vi "CreateSocketListener.vi"(0 "Universal Robot.lvclass in":refnum<class "Universal Robot.lvclass">, 5 "error in (no error)":errorcluster) -> (14 "Universal Robot.lvclass out":refnum<class "Universal Robot.lvclass">, 19 "error out":errorcluster)   [LabVIEW 2019, in "Universal Robot.lvclass"]
uses:
  Universal Robot.lvclass
  Universal Robot.lvclass/Universal Robot.ctl
  Client Interfaces/Socket Communication/Socket Communication.lvclass
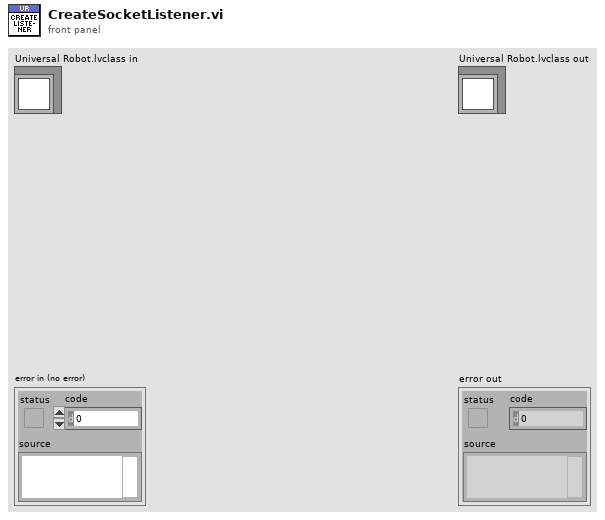
[diagram p1: front panel]
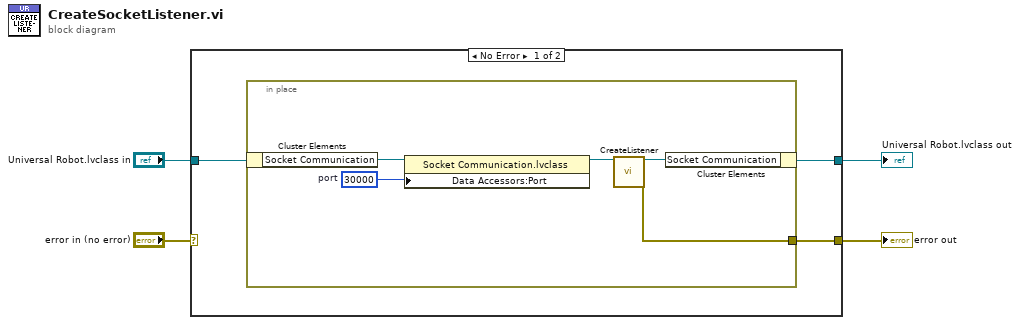
[diagram p0: block diagram]
diagram:
  n1 = case shown="No Error" "error in (no error)" {
    selector: "error in (no error)" -> [_ w14]
    tunnel: [w5 w14] -> w3
    tunnel: "Universal Robot.lvclass in" -> [w7 w13]
    tunnel: [w6 w13] -> w1
    frame No Error {
      n2 = in-place {
        in-place-border: [w9] -> w5
        w8 = u16 30000  # port
        n3 = in-place-cluster #1(w7) -> ("Socket Communication"=w12:refnum<class "Socket Communication.lvclass">)
        n4 = property class="Socket Communication.lvclass"(reference=w12, "Data Accessors:Port"=w8) -> (reference out=w11:refnum<class "Socket Communication.lvclass">)  [unwired: 1 in, 1 out]
        n5 = call "CreateListener.vi"("Socket Listener in"=w11) -> ("Socket Listener out"=w10:refnum<class "Socket Communication.lvclass">, "error out"=w9:errorcluster)  [unwired: 17 in]
        n6 = in-place-cluster #1("Socket Communication"=w10) -> (w6:refnum<class "Universal Robot.lvclass">)
      }
    }
    frame Error {
    }
  }
  "error out" <- w3
  "Universal Robot.lvclass out" <- w1
